vi "TranslatorBooster String Trim.vi"(9 "Count":u8, 11 "String In":string) -> (3 "Trimmed String":string)   [LabVIEW 2014, in "Complex Numbers.lvlib"]
uses:
  <vilib>/Aledyne-TSXperts/Arduino Compatible Compiler for LabVIEW/addons/Complex Numbers/Complex Numbers.lvlib
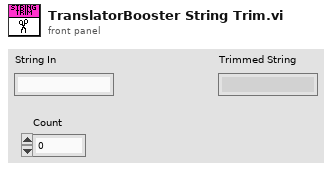
[diagram p1: front panel]
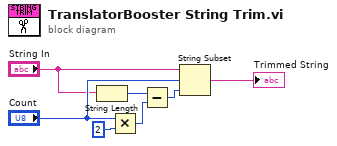
[diagram p0: block diagram]
diagram:
  n1 = String Length(string="String In") -> (length=w6:i32)
  n2 = Multiply(x="Count", y=u8 2) -> (x*y=w3:u8)
  n3 = Subtract(x=w6, y=w3) -> (x-y=w7:i32)
  n4 = String Subset(string="String In", offset (0)="Count", length (rest)=w7) -> (substring=→"Trimmed String":string)
